vi "LVClass_WavefrontCorrector Set WavefrontCorrectorSet.vi"(0 "WavefrontCorrector":refnum<class "WavefrontCorrector.lvclass">, 5 "WavefrontCorrectorSet":refnum<class "WavefrontCorrectorSet.lvclass">, 7 "load_and_apply_connection_params":bool, 9 "load_and_apply_params":bool, 11 "error in (no error)":errorcluster) -> (4 "WavefrontCorrector (dup)":refnum<class "WavefrontCorrector.lvclass">, 6 "WavefrontCorrectorSet (dup)":refnum<class "WavefrontCorrectorSet.lvclass">, 15 "error out":errorcluster)   [LabVIEW 2020, in "WavefrontCorrector.lvclass"]
doc: "Wavefront corrector parameter getter for parameter of type boolean.\n\n--------------------------------------------------------------------------------\n\n<B>correctorIn </B> : WavefrontCorrector object.\n<B>correctorOut </B> : WavefrontCorrector object.\n<B>parameter_name </B> : Name of the parameter.\n<B>value </B> : Value of the parameter.\n<B>ErrorIn </B> : Error\n<B>ErrorOut </B> : Error\n\n--------------------------------------------------------------------------------"
uses:
  WavefrontCorrector.lvclass
  WavefrontCorrectorSet.lvclass
  WavefrontCorrector.lvclass/WavefrontCorrector.ctl
  LVClass_WavefrontCorrectorSet Read WavefrontCorrectorSet.vi
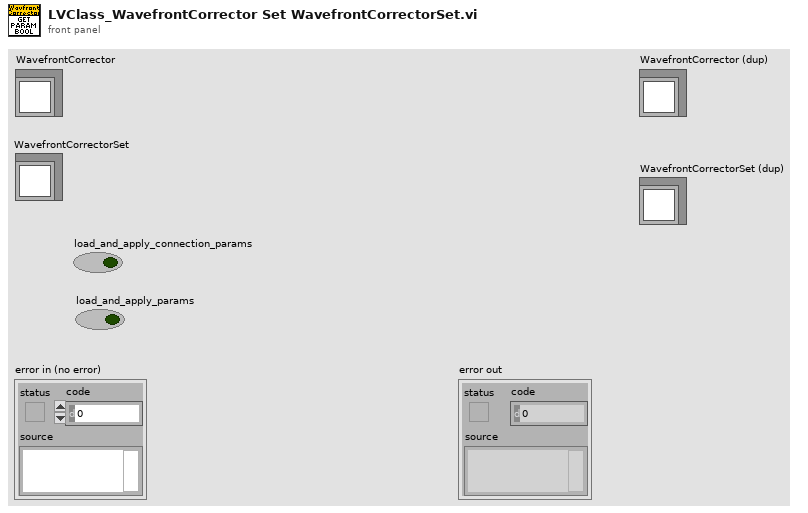
[diagram p1: front panel]
types:
  T1 = typedef "ClassID.ctl" = i64
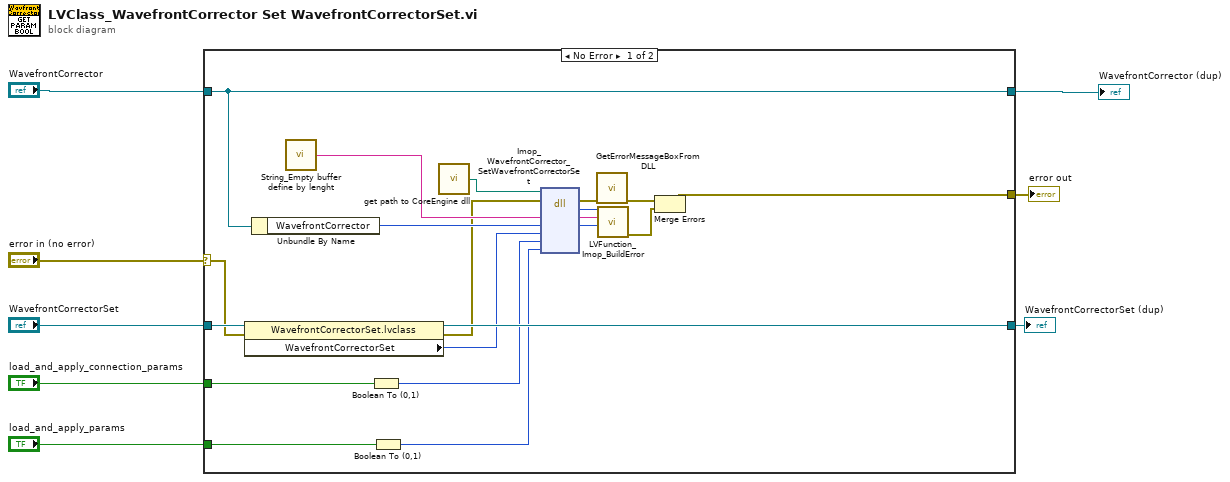
[diagram p0: block diagram]
diagram:
  n1 = case shown="No Error" "error in (no error)" {
    selector: "error in (no error)" -> [w17 w31]
    tunnel: [w15 w31] -> w6
    tunnel: [w20 w30] -> w5
    tunnel: "WavefrontCorrector" -> [w20 w30]
    tunnel: "WavefrontCorrectorSet" -> [w19 w29]
    tunnel: [w18 w29] -> w3
    tunnel: "load_and_apply_connection_params" -> [w13 _]
    tunnel: "load_and_apply_params" -> [w12 _]
    frame No Error {
      n2 = property class="WavefrontCorrectorSet.lvclass"(reference=w19, error in=w17) -> (reference out=w18:refnum<class "WavefrontCorrectorSet.lvclass">, error out=w16:errorcluster, "WavefrontCorrectorSet"=w14:T1)
      n3 = Unbundle By Name(w20) -> ("WavefrontCorrector"=w27:T1)
      n4 = call "String_Empty buffer define by lenght.vi"() -> ("Empty buffer"=w28:string)  [unwired: 1 in]
      n5 = Boolean To (0,1)(Boolean=w13) -> (0, 1=w11:i16)
      n6 = Boolean To (0,1)(Boolean=w12) -> (0, 1=w10:i16)
      n7 = call "get path to CoreEngine dll.vi"() -> ("path to wavekit library"=w24:path)  [unwired: 14 in, 1 out]
      n8 = dll-call lib="D:/soft/HASO_v3/SVN_trunk/ImOpCoreEngine4_LV2011/DLLs/c_interface_vc100.dll" fn="Imop_WavefrontCorrector_SetWavefrontCorrectorSet"(path in=w24, error in=w16, "message"=w28, "camera"=w27, "CameraSet"=w14, "load_and_apply_params"=w11, "load_and_apply_connection_params"=w10) -> (error out=w23:errorcluster, "return type"=w25:i32, "message"=w26:string, "camera"=w9:i64)  [unwired: 4 in, 1 out]
      n9 = call "GetErrorMessageBoxFromDLL.vi"("error IN"=w23) -> ("error OUT"=w22:errorcluster)  [unwired: 10 in]
      n10 = call "LVFunction_Imop_BuildError.vi"("code"=w25, "String to Prepend to source (\"\")"=w26, "Adresse"=w9) -> ("error out"=w21:errorcluster)  [unwired: 12 in]
      n11 = Merge Errors(w22, w21) -> (w15:errorcluster)
    }
    frame Error {
    }
  }
  "error out" <- w6
  "WavefrontCorrector (dup)" <- w5
  "WavefrontCorrectorSet (dup)" <- w3
